vi "UI.vi"() -> ()   [LabVIEW 2020]
uses:
  Controls/UI-Digital Pin.ctl
panel:
  in  "Stop":bool
  in  "Array":T1[](array[typedef]) {"Pin Value" format="%#_g V"}
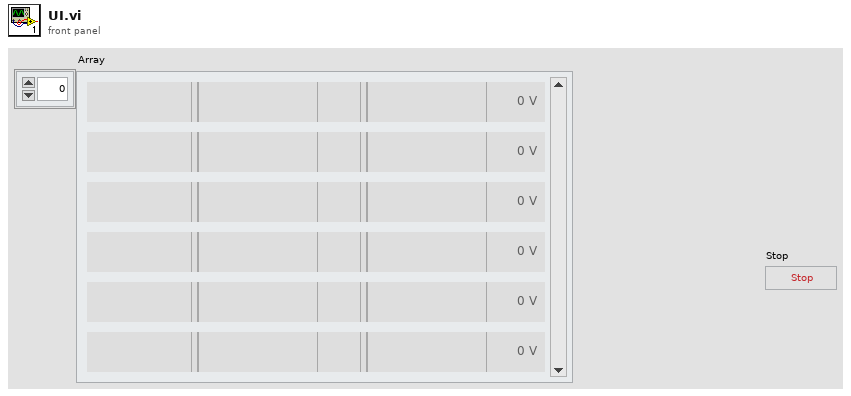
[diagram p1: front panel]
types:
  T1 = typedef "UI-Digital Pin.ctl" = cluster{"IO Direction":u16, "Pin Direction":string, "DO Value":u16, "Pin Value":dbl, "Pin Index":string, "Pin Mode":string}
  T2 = typedef "Transparent array.ctl" = T1[]
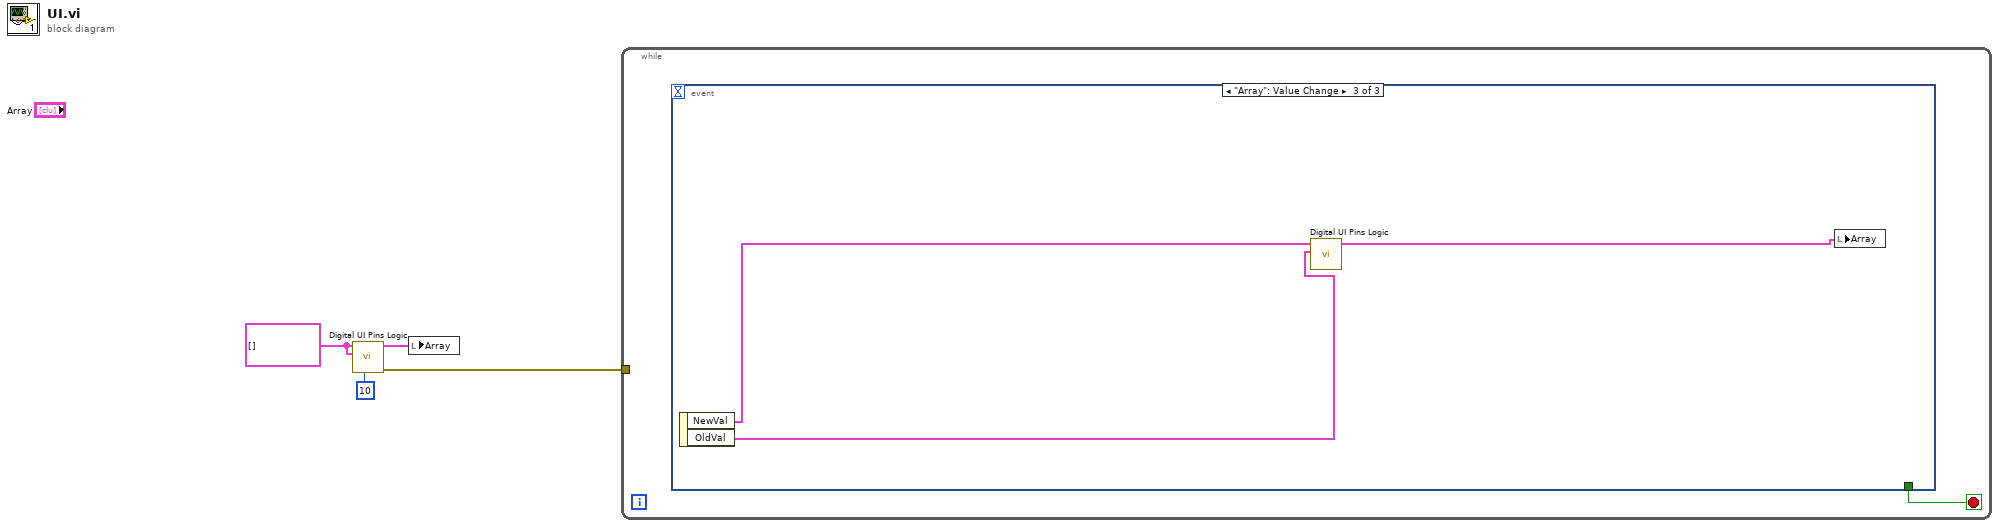
[diagram p0: block diagram]
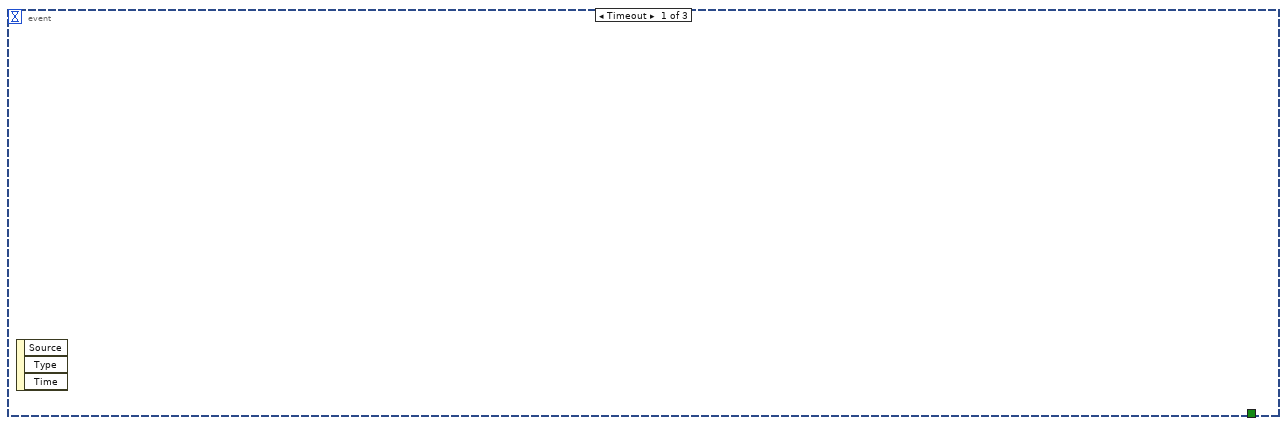
[diagram p2: hidden frame]
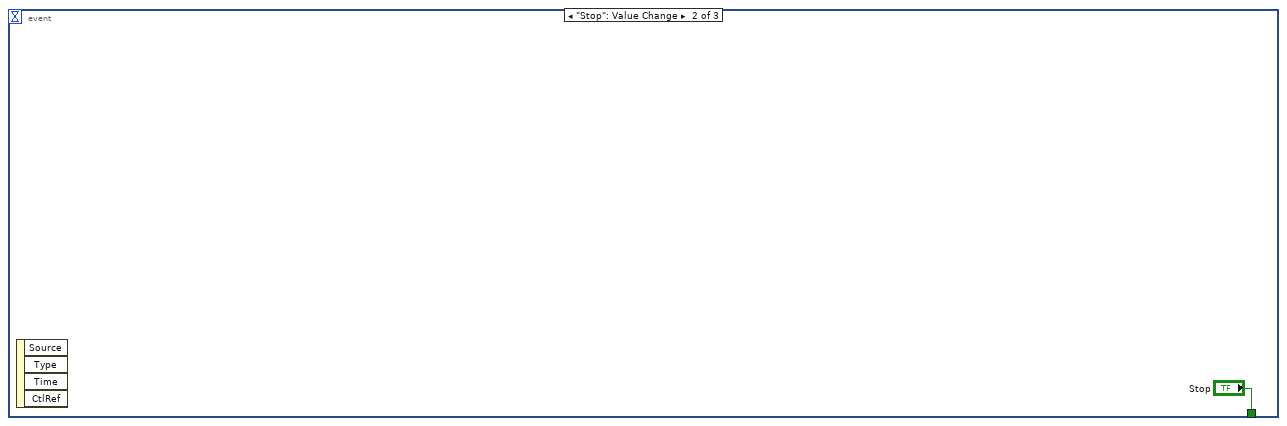
[diagram p3: hidden frame]
diagram:
  w2 = T1[] [] ("NewVal")
  n1 = call "Digital UI Pins Logic.vi"(6:10 ("Initial Array Size"), "OldVal"=w2, "NewVal"=w2) -> ("error out"=w1:errorcluster, "Updated Value"=w3:T2)  [unwired: 7 in]
  n2 = local write "Array"(w3) -> ()
  n3 = while {
    tunnel: w1 -> [_]
    stop <- w5 stop-if-true
    n4 = event shown="[2] \"Array\": Value Change" {
      selector: _ -> [_ _ _]
      dyn-events: _ -> [_ _ _]
      timeout: _ -> [_ _ _]
      tunnel: [_ "Stop" _] -> w5
      event Timeout {
        n5 = event-data() -> ()  [unwired: 1 in, 3 out]
      }
      event "Stop": Value Change {
        n6 = event-data() -> ()  [unwired: 1 in, 4 out]
      }
      event "Array": Value Change {
        n7 = event-data() -> ("NewVal"=w9:T1[], "OldVal"=w8:T1[])  [unwired: 1 in]
        n8 = call "Digital UI Pins Logic.vi"("OldVal"=w8, "NewVal"=w9) -> ("Updated Value"=w7:T2)  [unwired: 8 in, 1 out]
        n9 = local write "Array"(w7) -> ()
      }
    }
  }
